vi "1_PTLF_Classification_Training.vi"() -> ()   [LabVIEW 2020]
uses:
  <vilib>/Ngene/Deep Learning Toolkit/Toolkit/NN_Train/Controls/NN_LR_Policy_Cfg.ctl
  <vilib>/Ngene/Deep Learning Toolkit/Toolkit/NN_Train/Controls/NN_LR_Policy_Type.ctl
  <vilib>/Ngene/Deep Learning Toolkit/Toolkit/NN_Train/Controls/NN_Train_Session_Data.ctl
  <vilib>/Ngene/Deep Learning Toolkit/Toolkit/NN_Train/Controls/NN_Train_Params.ctl
  <vilib>/Ngene/Deep Learning Toolkit/Toolkit/NN_Train/Controls/NN_Train_Optimizer.ctl
  <vilib>/Ngene/Deep Learning Toolkit/Toolkit/NN_Train/Controls/NN_Train_Data_Sampling.ctl
  <vilib>/Ngene/Deep Learning Toolkit/Toolkit/NN_Network/Controls/NN_Device.ctl
  <vilib>/Ngene/Deep Learning Toolkit/Toolkit/NN_Layers/Layers/DropOut3D/Controls/NN_Layer_Config(DropOut3D).ctl
  <vilib>/Ngene/Deep Learning Toolkit/Toolkit/NN_Layers/Layers/Input/Controls/NN_Layer_Config_Aug(Input1D).ctl
  <vilib>/Ngene/Deep Learning Toolkit/Toolkit/NN_Layers/Layers/Input/Controls/Aug/NN_Input1D_Aug_Config.ctl
  <vilib>/Ngene/Deep Learning Toolkit/Toolkit/NN_Layers/Layers/Input/Controls/Aug/NN_Input1D_Aug_Types.ctl
  <vilib>/Ngene/Deep Learning Toolkit/Toolkit/NN_Layers/Layers/Input/Controls/Aug/Aug_Distribution_Type.ctl
  <vilib>/Ngene/Deep Learning Toolkit/Toolkit/NN_Network/Controls/NN_Save_Before_Destroy_Options.ctl
  <vilib>/Ngene/Deep Learning Toolkit/Toolkit/NN_Layers/Layers/FC/Controls/NN_Layer_Config(FC).ctl
  <vilib>/Ngene/Deep Learning Toolkit/Toolkit/NN_Layers/Layers/BatchNorm/Controls/NN_BN_Params.ctl
  <vilib>/Ngene/Deep Learning Toolkit/Toolkit/NN_Activations/Controls/NN_Activation_Type.ctl
  <vilib>/Ngene/Deep Learning Toolkit/Toolkit/NN_Layers/Controls/NN_Layer_Init_Params.ctl
  <vilib>/Ngene/Deep Learning Toolkit/Toolkit/NN_Layers/Controls/NN_Layer_Weight_Init_Type.ctl
  <vilib>/Ngene/Deep Learning Toolkit/Toolkit/NN_Layers/Layers/Input/Controls/NN_Layer_Config(Input1D).ctl
  <vilib>/Ngene/Deep Learning Toolkit/Toolkit/NN_Data/Controls/NN_Data_type.ctl
  <vilib>/Ngene/Deep Learning Toolkit/Toolkit/NN_Layers/Layers/Input/NN_Layer_Create(Input1D).vi
  <vilib>/Ngene/Deep Learning Toolkit/Toolkit/NN_Layers/Layers/FC/NN_Layer_Create(FC).vi
  <vilib>/Ngene/Deep Learning Toolkit/Toolkit/NN_Layers/Layers/Dropout/NN_Layer_Create(DropOut).vi
  <vilib>/Ngene/Deep Learning Toolkit/Toolkit/NN_Layers/Layers/SoftMax/NN_Layer_Create(SoftMax).vi
  <vilib>/Ngene/Deep Learning Toolkit/Toolkit/NN_Train/Loss_Functions/NN_Set_Loss(CrossEntropy).vi
  <vilib>/Ngene/Deep Learning Toolkit/Toolkit/NN_Network/subVIs/NN_Predict/NN_Predict(In1D_Out1D).vi
  <vilib>/Ngene/Deep Learning Toolkit/Toolkit/NN_Train/Eval_Loss/NN_Eval_Test_Error_Loss/NN_Eval(In1D_Out1D).vi
  <vilib>/Ngene/Deep Learning Toolkit/Toolkit/NN_Train/Eval_Loss/NN_Calc_Cofusion_Matrix/NN_Calc_Confusion_Matrix(In1D_Out1D).vi
  <vilib>/Ngene/Deep Learning Toolkit/Toolkit/Deep_Learning_Toolkit_by_Ngene.lvlib
  <vilib>/ptbypt/NI_PtbyPt.lvlib
panel:
  in  "Tab Control":enum32{"Training", "Evaluation"}(tab)
  in  "Working Dir":path=path "D:/Ngene/Projects_SVN/DeepLTK_FPGA/Projects/Examples/3_PTLF_Classification(PXI,sbRIO)/Models/0_PTLF_Classification_Original"
  in  "LR Update Policy":T1={"Policy_Type"=enum."Step", "LR0"=0.0001, "k"=30.0, "WarmUp_Policy"=enum."Ramp", "WarmUp_Iter"=1000, "WarmUp_Ratio"=10.0} {"WarmUp_Ratio" min=1; "WarmUp_Iter" min=1; "LR0" format="%.7f"}
  out "Session Data":T3={"Epochs"=114.948265, "Tot_Iter"=26941, "LR"=1.25e-05, "LR_iter"=26942}
  in  "NN_Train_Params":T4={"Optimizer"=enum."Adam", "Beta_1"=0.9, "Beta_2"=0.999, "Weight Decay(L1)"=7e-07, "Weight Decay(L2)"=7e-07, "Data_Sampling"=enum."Random"}
  in  "Stop Training":bool
  out "Test Error":sgl
  out "Test Loss":sgl
  in  "NN_Device":T7
  out "Loss Graphs":cluster{"mean":dbl, "mean":dbl, "mean":dbl}(graph)={"mean"=0.06423647763207554, "mean"=0.039573706686496735, "mean"=0.013333333656191826}
  in  "Eval":bool
  out "Training Loss":sgl
  in  "Train dataset path":path=path "D:/Ngene/Projects_SVN/DeepLTK_FPGA/Projects/Examples/3_PTLF_Classification(PXI,sbRIO)/Dataset/Train"
  in  "Test dataset path":path=path "D:/Ngene/Projects_SVN/DeepLTK_FPGA/Projects/Examples/3_PTLF_Classification(PXI,sbRIO)/Dataset/Test"
  out "Time_Elapsed":dbl=158.89084720000005 format="%<%H:%M:%S>t"
  out "Confusion Matrix":string[][](table)=[["200", "0", "0", "0", "0", "0", "1.0000"], ["0", "200", "0", "0", "0", "0", "1.0000"], ["0", "0", "200", "0", "0", "0", "1.0000"], ["0", "0", "0", "200", "0", "0", "1.0000"], ["0", "0", "0", "15", "185", "0", "0.9250"], ["0", "0", "1", "0", "0", "199", "0.9950"], ["1.0000", "1.0000", "0.9950", "0.9302", "1.0000", "1.0000", ""]]
  # "Overview: This example demonstrating the usage of Deep Learning Toolkit for solving  Power Transmission Line Fault classification problem.\nRequirements: DeepLTK - Deep Learning Toolkit for LabVIEW (https://www.ngene.co/deep-learning-toolkit-for-labview)\nInstructions:\n1.\tSpecify the paths to the Train and Test datasets in the \"Train Dataset Path\" and \"Test Dataset Path\" fields, respectively.\n2.\tRun the VI with current configuration of the training parameters and Learning Rate update policy.\n3.\tObserve how the training loss is decreasing.\n4.\tWait about 2 minutes and press the \"Stop\" button when the loss is not decreasing anymore.\nMore Examples: https://github.com/ngenehub/deepltk_fpga_examples"
  # "Power Transmission Line Fault Classification - Training"
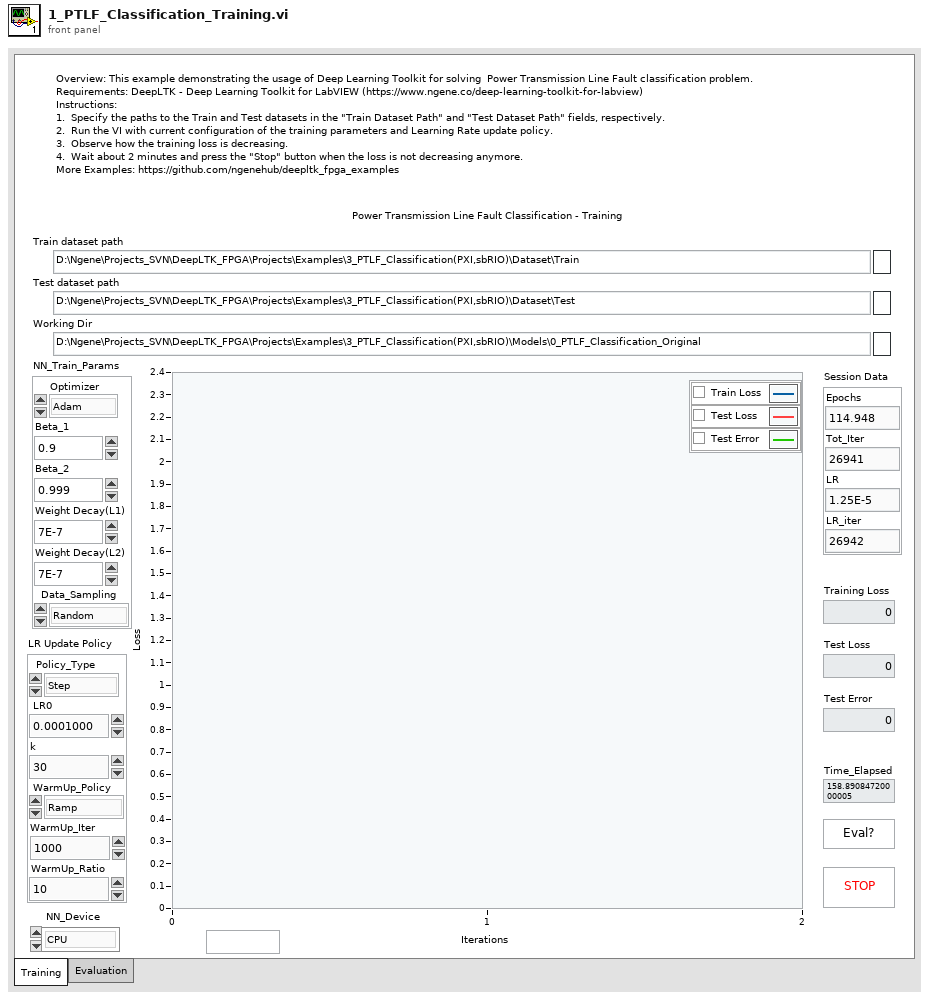
[diagram p1: front panel]
types:
  T1 = typedef "Deep_Learning_Toolkit_by_Ngene.lvlib/NN_LR_Policy_Cfg.ctl" = cluster{"Policy_Type":T2, "LR0":dbl, "k":sgl, "WarmUp_Policy":enum16{"Step", "Ramp"}, "WarmUp_Iter":i32, "WarmUp_Ratio":sgl}
  T2 = typedef "Deep_Learning_Toolkit_by_Ngene.lvlib/NN_LR_Policy_Type.ctl" = enum16{"Manual", "Step", "Exp", "1/t"}
  T3 = typedef "Deep_Learning_Toolkit_by_Ngene.lvlib/NN_Train_Session_Data.ctl" = cluster{"Epochs":sgl, "Tot_Iter":i32, "LR":sgl, "LR_iter":i32}
  T4 = typedef "Deep_Learning_Toolkit_by_Ngene.lvlib/NN_Train_Params.ctl" = cluster{"Optimizer":T5, "Beta_1":sgl, "Beta_2":sgl, "Weight Decay(L1)":sgl, "Weight Decay(L2)":sgl, "Data_Sampling":T6}
  T5 = typedef "Deep_Learning_Toolkit_by_Ngene.lvlib/NN_Train_Optimizer.ctl" = enum16{"SGD", "Adam", "Adagrad", "Adadelta", "RMSProp", "Nesterov"}
  T6 = typedef "Deep_Learning_Toolkit_by_Ngene.lvlib/NN_Train_Data_Sampling.ctl" = enum16{"Random", "Sequential"}
  T7 = typedef "Deep_Learning_Toolkit_by_Ngene.lvlib/NN_Device.ctl" = enum16{"CPU", "GPU"}
  T8 = typedef "Deep_Learning_Toolkit_by_Ngene.lvlib/NN_Layer_Config(DropOut3D).ctl" = cluster{"Name":string, "Probability":sgl}
  T9 = typedef "Deep_Learning_Toolkit_by_Ngene.lvlib/NN_Layer_Config_Aug(Input1D).ctl" = T10[]
  T10 = typedef "Deep_Learning_Toolkit_by_Ngene.lvlib/NN_Input1D_Aug_Config.ctl" = cluster{"Aug Type(1D)":T11, "Aug Value":sgl, "Distribution":T12}
  T11 = typedef "Deep_Learning_Toolkit_by_Ngene.lvlib/NN_Input1D_Aug_Types.ctl" = enum16{"Add_Noise", "Mult_Noise", "Shift", "Scale"}
  T12 = typedef "Deep_Learning_Toolkit_by_Ngene.lvlib/Aug_Distribution_Type.ctl" = enum16{"Uniform", "Gaussian"}
  T13 = typedef "Deep_Learning_Toolkit_by_Ngene.lvlib/NN_Save_Before_Destroy_Options.ctl" = cluster{"CFG?":bool, "Weights?":bool, "Render?":bool}
  T14 = typedef "Deep_Learning_Toolkit_by_Ngene.lvlib/NN_Layer_Config(FC).ctl" = cluster{"Name":string, "Size":i32, "BN":bool, "BN_Params":T15, "Activation":T16, "Has Bias?":bool, "Init_Params":T17, "Custom_Params":string}
  T15 = typedef "Deep_Learning_Toolkit_by_Ngene.lvlib/NN_BN_Params.ctl" = cluster{"epsilon":sgl, "momentum":sgl}
  T16 = typedef "Deep_Learning_Toolkit_by_Ngene.lvlib/NN_Activation_Type.ctl" = enum16{"Sigmoid", "ReLU", "LReLU", "ReLU6", "tanh", "Swish", "Mish", "None"}
  T17 = typedef "Deep_Learning_Toolkit_by_Ngene.lvlib/NN_Layer_Init_Params.ctl" = cluster{"Init_Type":T18, "Value":sgl}
  T18 = typedef "Deep_Learning_Toolkit_by_Ngene.lvlib/NN_Layer_Weight_Init_Type.ctl" = enum16{"Const", "Uniform", "Gaussian", "Xavier"}
  T19 = typedef "Deep_Learning_Toolkit_by_Ngene.lvlib/NN_Layer_Config(Input1D).ctl" = cluster{"Name":string, "Size":i32, "Data_Type":T20, "Shift":sgl, "Scale":sgl}
  T20 = typedef "Deep_Learning_Toolkit_by_Ngene.lvlib/NN_Data_type.ctl" = enum16{"I8", "U8", "I16", "U16", "U32 ARGB", "SGL"}
  T21 = typedef "Deep_Learning_Toolkit_by_Ngene.lvlib/NN_DataSets_All(In1D_Out1D).ctl" = cluster{"Train":T22, "Validation":T22, "Test":T22}
  T22 = typedef "Deep_Learning_Toolkit_by_Ngene.lvlib/NN_DataSet(In1D_Out1D).ctl" = cluster{"Inputs Ref.":variant, "Outputs Ref.":T23, "Dims_In":i32, "Dataset_Size":i32, "Dims_Out":i32, "Labels":string[], "File Paths":path[]}
  T23 = typedef "Deep_Learning_Toolkit_by_Ngene.lvlib/NN_Data_ref(2D_SGL).ctl" = refnum<data-value>
  T24 = typedef "Deep_Learning_Toolkit_by_Ngene.lvlib/NN.ctl" = cluster{"Name":string, "No of Layers":i32, "mBatch":i32, "Layers":T25[], "Dimty":T26, "Dims_In":T27, "Dims_Out":T27, "Working_Dir":path, "Train?":bool, "Train_Params":T4, "LR_Update_Policy":T1, "Session Data":T3, "Ground_truth":T28, "NNg_hdls":T29, "NN_Device":T7, "GPU Id":i32, "Labels":string[], "Receptive Field":T30[], "Loss_Type":T31, "Loss_Cfg_Prms":variant, "NNG_WS":T32}
  T25 = typedef "Deep_Learning_Toolkit_by_Ngene.lvlib/NN_Layer_ref.ctl" = refnum<data-value>
  T26 = typedef "Deep_Learning_Toolkit_by_Ngene.lvlib/NN_In_Out_Dim-ty.ctl" = enum8{"In1D_Out1D", "In3D_Out1D", "In3D_Out3D", "In3D_OutBBox"}
  T27 = typedef "Deep_Learning_Toolkit_by_Ngene.lvlib/NN_Dims(C,H,W).ctl" = cluster{"C":i32, "H":i32, "W":i32}
  T28 = typedef "Deep_Learning_Toolkit_by_Ngene.lvlib/NN_Ground_truth.ctl" = cluster{"Y":variant}
  T29 = typedef "Deep_Learning_Toolkit_by_Ngene.lvlib/nng_cuda_handles.ctl" = cluster{"cudnn":u64, "cublas":u64, "stream":u64, "curand":u64}
  T30 = typedef "Deep_Learning_Toolkit_by_Ngene.lvlib/NN_Dims(V,H).ctl" = cluster{"V":i32, "H":i32}
  T31 = typedef "Deep_Learning_Toolkit_by_Ngene.lvlib/NN_Loss_Type.ctl" = enum16{"None", "MSE", "CrossEntropy", "YOLO_v2", "YOLO_v4"}
  T32 = typedef "Deep_Learning_Toolkit_by_Ngene.lvlib/NNG_WS.ctl" = cluster{"NNG_WS_Mem":T33, "Max_WS_Size":i64}
  T33 = typedef "Deep_Learning_Toolkit_by_Ngene.lvlib/NNg_WS_Mem_DVR.ctl" = refnum<data-value>
  T34 = typedef "Deep_Learning_Toolkit_by_Ngene.lvlib/NN_Eval_Params.ctl" = cluster{"Loss":sgl, "Error":sgl}
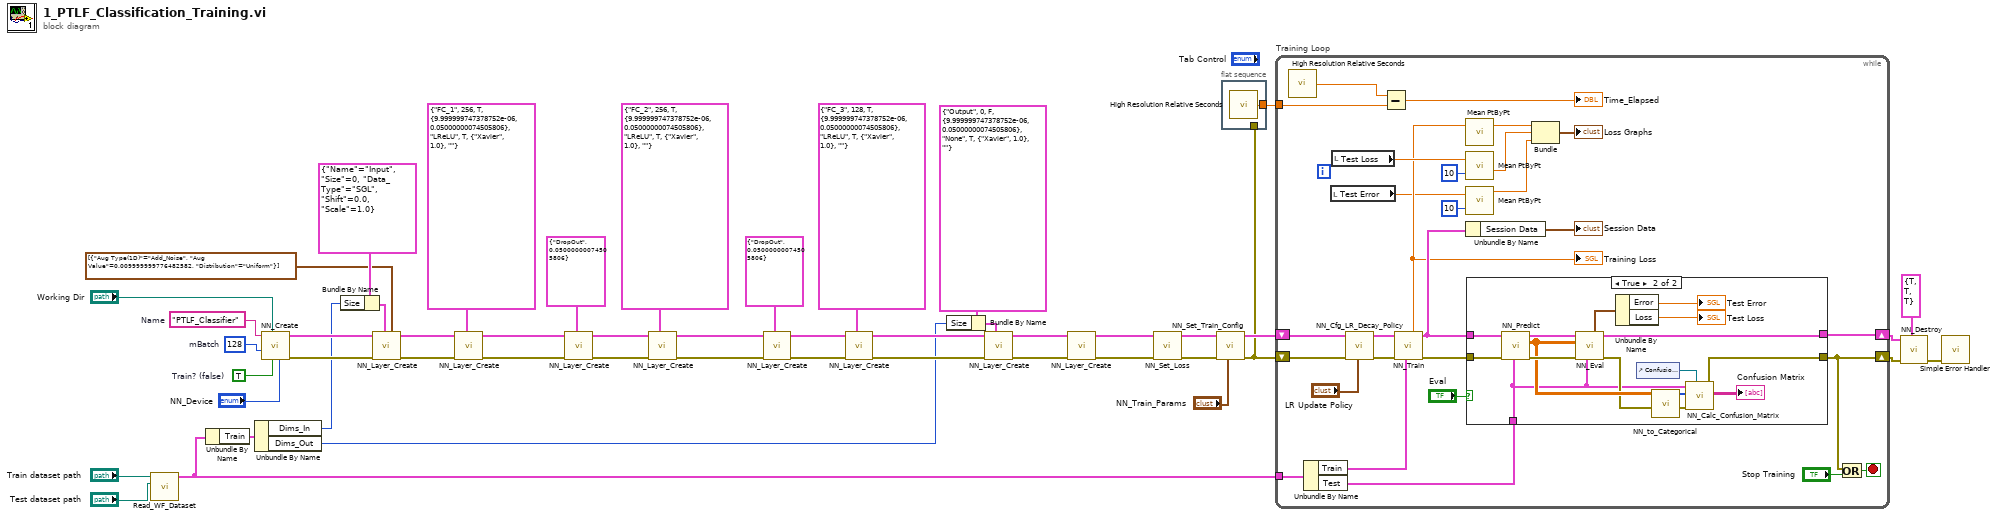
[diagram p0: block diagram]
diagram:
  w33 = "PTLF_Classifier"  # Name
  w34 = 128  # mBatch
  w35 = TRUE  # Train? (false)
  n1 = call "Read_WF_Dataset.vi"("Test dataset path"="Test dataset path", "Train dataset path"="Train dataset path") -> ("NN_Dataset"=w18:T21)  [unwired: 9 in]
  n2 = Unbundle By Name(w18) -> ("Train"=w3:T22)
  n3 = Unbundle By Name(w3) -> ("Dims_In"=w19:i32, "Dims_Out"=w2:i32)
  n4 = call <vilib>:"NN_Create.vi"("NN_Device"="NN_Device", "Train? (false)"=w35, "Working Dir"="Working Dir", "mBatch (1)"=w34, "Name"=w33) -> ("error out"=w48:errorcluster, "NN out"=w49:T24)  [unwired: 5 in]
  n5 = Bundle By Name(cluster=T19 {"Name"="Input", "Size"=0, "Data_Type"=enum."SGL", "Shift"=0.0, "Scale"=1.0} ("Input1D_Cfg"), "Size"=w19) -> (w40:T19)
  n6 = call-poly <vilib>:"NN_Layer_Create.vi"("Aug Config Params(1D)"=T9 [{"Aug Type(1D)"=enum."Add_Noise", "Aug Value"=0.01, "Distribution"=enum."Uniform"}], "Input1D_Cfg"=w40, "error in (no error)"=w48, "NN in"=w49) -> ("error out"=w37:errorcluster, "NN out"=w38:T24)  [unwired: 5 in, 1 out]
  n7 = call-poly <vilib>:"NN_Layer_Create.vi"("FC_Cfg"=T14 {"Name"="FC_1", "Size"=256, "BN"=TRUE, "BN_Params"={"epsilon"=1e-05, "momentum"=0.05}, "Activation"=enum."LReLU", "Has Bias?"=TRUE, "Init_Params"={"Init_Type"=enum."Xavier", "Value"=1.0}, "Custom_Params"=""} ("FC_Cfg_1"), "error in (no error)"=w37, "NN in"=w38) -> ("error out"=w8:errorcluster, "NN out"=w9:T24)  [unwired: 6 in, 1 out]
  n8 = call-poly <vilib>:"NN_Layer_Create.vi"("DropOut_Cfg"=T8 {"Name"="DropOut", "Probability"=0.05}, "error in (no error)"=w8, "NN in"=w9) -> ("error out"=w6:errorcluster, "NN out"=w7:T24)  [unwired: 6 in, 1 out]
  n9 = call-poly <vilib>:"NN_Layer_Create.vi"("FC_Cfg"=T14 {"Name"="FC_2", "Size"=256, "BN"=TRUE, "BN_Params"={"epsilon"=1e-05, "momentum"=0.05}, "Activation"=enum."LReLU", "Has Bias?"=TRUE, "Init_Params"={"Init_Type"=enum."Xavier", "Value"=1.0}, "Custom_Params"=""} ("FC_Cfg_1"), "error in (no error)"=w6, "NN in"=w7) -> ("error out"=w11:errorcluster, "NN out"=w14:T24)  [unwired: 6 in, 1 out]
  n10 = call-poly <vilib>:"NN_Layer_Create.vi"("DropOut_Cfg"=T8 {"Name"="DropOut", "Probability"=0.05}, "error in (no error)"=w11, "NN in"=w14) -> ("error out"=w12:errorcluster, "NN out"=w13:T24)  [unwired: 6 in, 1 out]
  n11 = call-poly <vilib>:"NN_Layer_Create.vi"("FC_Cfg"=T14 {"Name"="FC_3", "Size"=128, "BN"=TRUE, "BN_Params"={"epsilon"=1e-05, "momentum"=0.05}, "Activation"=enum."LReLU", "Has Bias?"=TRUE, "Init_Params"={"Init_Type"=enum."Xavier", "Value"=1.0}, "Custom_Params"=""} ("FC_Cfg_1"), "error in (no error)"=w12, "NN in"=w13) -> ("error out"=w24:errorcluster, "NN out"=w25:T24)  [unwired: 6 in, 1 out]
  n12 = Bundle By Name(cluster=T14 {"Name"="Output", "Size"=0, "BN"=FALSE, "BN_Params"={"epsilon"=1e-05, "momentum"=0.05}, "Activation"=enum."None", "Has Bias?"=TRUE, "Init_Params"={"Init_Type"=enum."Xavier", "Value"=1.0}, "Custom_Params"=""} ("FC_Cfg_1"), "Size"=w2) -> (w39:T14)
  n13 = call-poly <vilib>:"NN_Layer_Create.vi"("FC_Cfg"=w39, "error in (no error)"=w24, "NN in"=w25) -> ("error out"=w43:errorcluster, "NN out"=w44:T24)  [unwired: 6 in, 1 out]
  n14 = call-poly <vilib>:"NN_Layer_Create.vi"("error in (no error)"=w43, "NN in"=w44) -> ("error out"=w30:errorcluster, "NN out"=w45:T24)  [unwired: 7 in, 1 out]
  n15 = call-poly <vilib>:"NN_Set_Loss.vi"("error in (no error)"=w30, "NN in"=w45) -> ("error out"=w29:errorcluster, "NN out"=w31:T24)  [unwired: 8 in]
  n16 = call <vilib>:"NN_Set_Train_Config.vi"("NN_Train_Params"="NN_Train_Params", "error in (no error)"=w29, "NN in"=w31) -> ("error out"=w16:errorcluster, "NN out"=w36:T24)  [unwired: 7 in]
  n17 = flat-sequence {
    tunnel: w16 -> [_]
    tunnel: [w50] -> w15
    frame #0 {
      n18 = call <vilib>:"High Resolution Relative Seconds.vi"() -> ("relative seconds"=w50:dbl)
    }
  }
  n19 = while "Training Loop" {
    shift-right: [w63] -> w22
    shift-left: w16 -> [w73]
    shift-right: [w69] -> w23
    shift-left: w36 -> [w76]
    tunnel: w18 -> [w59]
    tunnel: w15 -> [w57]
    stop <- w64 stop-if-true
    n20 = call <vilib>:"High Resolution Relative Seconds.vi"() -> ("relative seconds"=w56:dbl)
    n21 = Unbundle By Name(w59) -> ("Train"=w51:T22, "Test"=w58:T22)
    n22 = local read "Test Error"() -> (w53:sgl)
    n23 = local read "Test Loss"() -> (w67:sgl)
    n24 = call <vilib>:"NN_Cfg_LR_Decay_Policy.vi"("LR_Decay_Params"="LR Update Policy", "error in (no error)"=w73, "NN in"=w76) -> ("error out"=w74:errorcluster, "NN out"=w75:T24)  [unwired: 7 in]
    n25 = Subtract(x=w56, y=w57) -> (x-y=→"Time_Elapsed":dbl)
    n26 = call <vilib>:"NN_Train.vi"("Train Dataset"=w51, "error in (no error)"=w74, "NN in"=w75) -> ("error out"=w70:errorcluster, "NN out"=w71:T24, "Loss"=w65:sgl)  [unwired: 3 in, 3 out]
    "Training Loss" <- w65
    n27 = call <vilib>:"Mean PtByPt.vi"("x"=w65) -> ("mean"=w61:dbl)  [unwired: 3 in, 1 out]
    n28 = call <vilib>:"Mean PtByPt.vi"("x"=w67, "sample length"=10) -> ("mean"=w62:dbl)  [unwired: 2 in, 1 out]
    n29 = call <vilib>:"Mean PtByPt.vi"("x"=w53, "sample length"=10) -> ("mean"=w52:dbl)  [unwired: 2 in, 1 out]
    n30 = Unbundle By Name(w71) -> ("Session Data"=→"Session Data":T3)
    n31 = case shown="True" "Eval" {
      tunnel: w71 -> [w80 w94]
      tunnel: w70 -> [w79 w93]
      tunnel: [w80 w92] -> w69
      tunnel: [w79 w87] -> w63
      tunnel: w58 -> [_ w84]
      frame False {
      }
      frame True {
        n32 = call-poly <vilib>:"NN_Predict.vi"("Dataset"=w84, "error in (no error)"=w93, "NN in"=w94) -> ("error out"=w95:errorcluster, "Predictions"=w90:sgl[][], "NN out"=w91:T24)  [unwired: 6 in]
        n33 = call-poly <vilib>:"NN_Eval.vi"("Dataset"=w84, "error in (no error)"=w95, "Predictions"=w90, "NN in"=w91) -> ("error out"=w88:errorcluster, "NN out"=w92:T24, "NN_Eval_Params"=w83:T34)  [unwired: 4 in, 1 out]
        n34 = Unbundle By Name(w83) -> ("Error"=→"Test Error":sgl, "Loss"=→"Test Loss":sgl)
        n35 = control-ref of="Confusion Matrix"() -> (w85:refnum<vi>)
        n36 = call <vilib>:"NN_to_Categorical.vi"("Prediction"=w90) -> ("Label_Idx"=w89:i32[])  [unwired: 10 in]
        n37 = call-poly <vilib>:"NN_Calc_Confusion_Matrix.vi"("Confusion Matrix (Table) ref."=w85, "error in (no error)"=w88, "Predictions"=w89, "Dataset"=w84) -> ("error out"=w87:errorcluster, "Confusion Matrix (Table)"=→"Confusion Matrix":string[][])  [unwired: 3 in, 3 out]
      }
    }
    n38 = Bundle("mean"=w61, "mean"=w62, "mean"=w52) -> (→"Loss Graphs":cluster{"mean":dbl, "mean":dbl, "mean":dbl})  [unwired: 1 in]
    n39 = Or(x=w63, y="Stop Training") -> (x .or. y?=w64:bool)
  }
  n40 = call <vilib>:"NN_Destroy.vi"("Save (T, T, T)"=T13 {"CFG?"=TRUE, "Weights?"=TRUE, "Render?"=TRUE}, "error in (no error)"=w22, "NN in"=w23) -> ("error out"=w42:errorcluster)  [unwired: 7 in, 1 out]
  n41 = call <vilib>:"Simple Error Handler.vi"("error in (no error)"=w42) -> ()  [unwired: 4 in, 5 out]
